vi "add_download_location.vi"(8 "error in (no error)":errorcluster, 11 "path":path) -> (0 "error out":errorcluster)   [LabVIEW 2015, in "lv-post-installer.lvlib"]
uses:
  lv-post-installer.lvlib
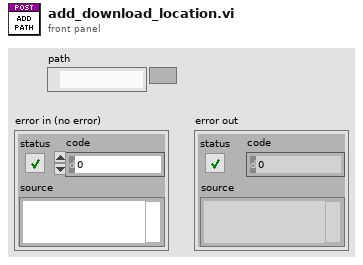
[diagram p1: front panel]
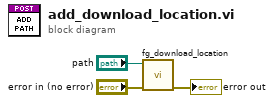
[diagram p0: block diagram]
diagram:
  n1 = call "fg_download_location.vi"("error in (no error)"="error in (no error)", "path in"="path") -> ("error out"=→"error out":errorcluster)  [unwired: 8 in, 1 out]
